vi "FPGA.vi"() -> ()   [LabVIEW 2013]
uses:
  <vilib>/rvi/FXPMathLib/FxpSinAndCos/XNode/nifxpmath_SinAndCos.xnode
  <vilib>/eio/EIONode/EIONode.xnode
  <vilib>/rvi/eio/common/nirviEmuTemplateMethod_errors.vi
  ToFPGA.ctl
  <vilib>/rvi/FXPMathLib/FxpSinAndCos/simVIs/DllFxpSinAndCosTemp_sub.vi
  <vilib>/rvi/FXPMathLib/FxpSinAndCos/subVIs/nifxpmath_SinAndCos_SimConfig.ctl
  FreqEstimator.ctl
  PMUmeasurements.ctl
panel:
  in  "Hold Time":sgl
  out "Loop period monitoring":u8
  out "output cluster":T1
  out "FPGA Error Out":errorcluster
  in  "alpha_Load":sgl
  in  "Scaling":sgl=80.0
  in  "Frequency Estimator Settings":T2={"Parameters"={"Ts"=5e-05, "kappaav"=0.625, "kappaph"=0.5762, "mu"=0.7086}}
  in  "Freq of Osc Load":sgl=0.64
  in  "PMU measurments":T3
  in  "stop":bool
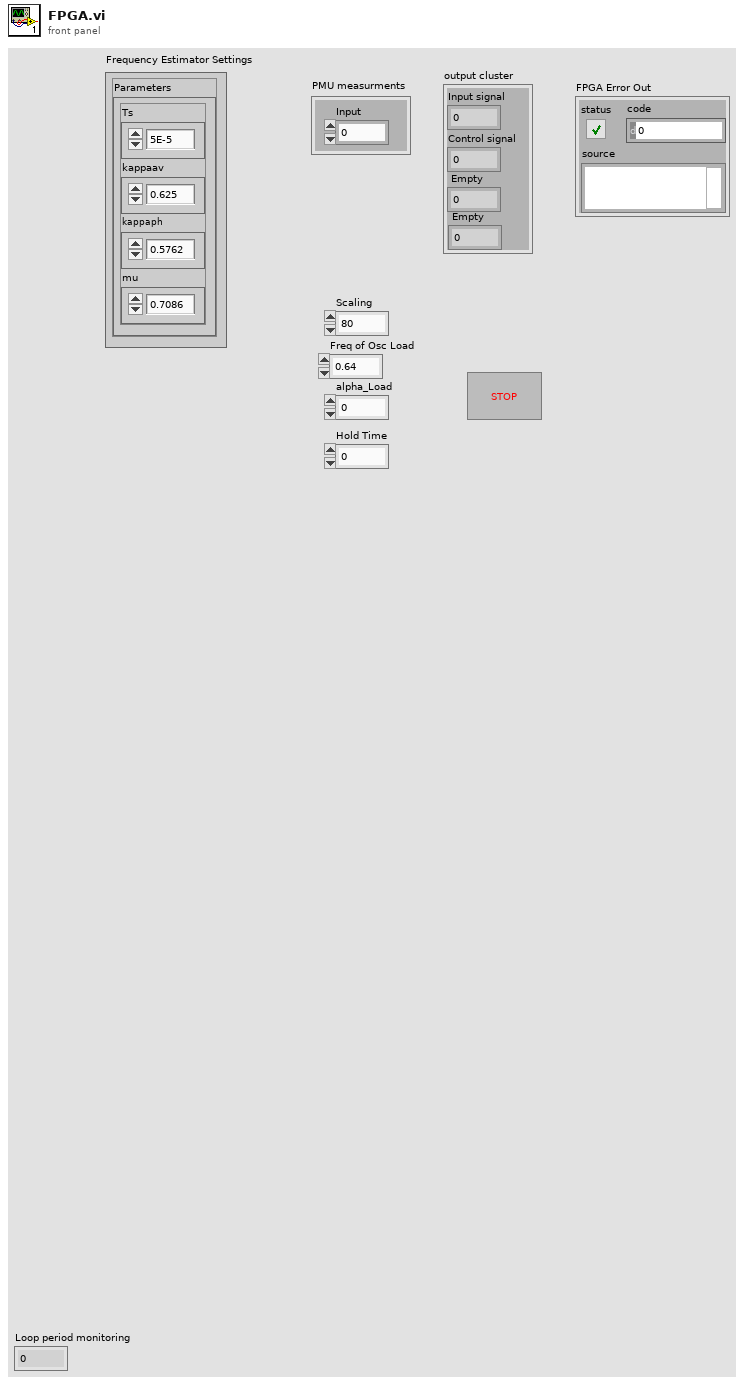
[diagram p1: front panel]
types:
  T1 = typedef "ToFPGA.ctl" = cluster{"Input signal":sgl, "Control signal":sgl, " Empty":sgl, " Empty":sgl}
  T2 = typedef "FreqEstimator.ctl" = cluster{"Parameters":cluster{"Ts":sgl, "kappaav":sgl, "kappaph":sgl, "mu":sgl}}
  T3 = typedef "PMUmeasurements.ctl" = cluster{"Input":sgl}
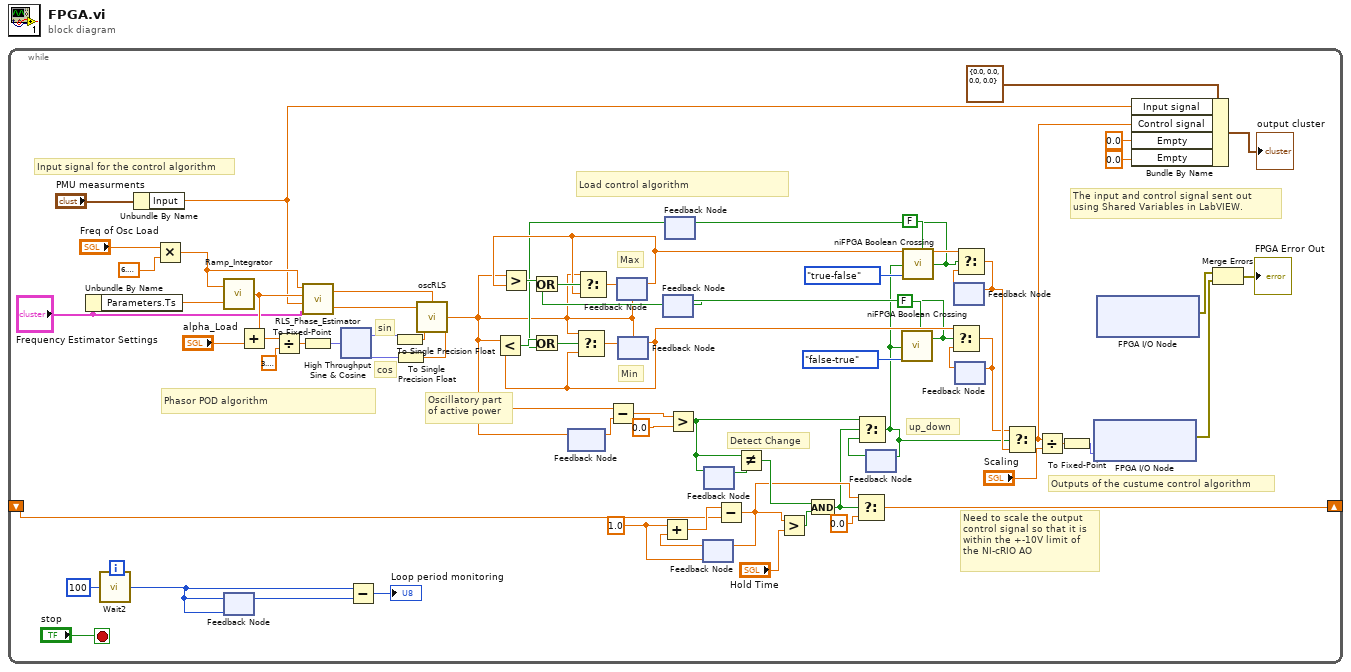
[diagram p0: block diagram]
diagram:
  n1 = while {
    shift-right: [w31] -> _
    shift-left: _ -> [w30]
    stop <- "stop" stop-if-true
    w37 = sgl 1.0 ("y")
    # "Need to scale the output \ncontrol signal so that it is \nwithin the +-10V limit of \nthe NI-cRIO AO"
    # "Load control algorithm"
    # "Phasor POD algorithm"
    # "Input signal for the control algorithm"
    # "The input and control signal sent out using Shared Variables in LabVIEW."
    # "Outputs of the custume control algorithm"
    # "up_down"
    # "Detect Change"
    # "Min"
    # "Max"
    # "Oscillatory part \nof active power"
    # "cos"
    # "sin"
    n2 = Unbundle By Name("Frequency Estimator Settings") -> ("Parameters.Ts"=w9:sgl)
    n3 = call "Wait2"("Count(uSec)"=u8 100) -> ("Tick Count(uSec)"=w41:u8)
    n4 = Unbundle By Name("PMU measurments") -> ("Input"=w7:sgl)
    n5 = Multiply(x="Freq of Osc Load", y=sgl 6.2831855) -> (x*y=w69:sgl)
    n6 = call "Ramp_Integrator.vi"("tsample"=w9, "w"=w69) -> ("theta"=w49:sgl)
    n7 = feedback #1(w41) -> (w42:u8)
    n8 = feedback-in #1(w41) -> ()
    n9 = Add(x=w49, y="alpha_Load") -> (x+y=w48:sgl)
    n10 = Divide(x=w48, y=sgl 3.1415927) -> (x/y=w67:sgl)
    n11 = call "RLS_Phase_Estimator.vi"("Frequency Estimator Settings"="Frequency Estimator Settings", "u"=w7, "theta"=w49, "wcs"=w69) -> ("uphq"=w60:sgl, "uphd"=w61:sgl)
    n12 = To Fixed-Point(number=w67) -> (fixed-point=w66:fxp<+/-,20,5>)  [unwired: 1 in]
    n13 = xnode "High Throughput Sine & Cosine"("x (pi)"=w66) -> ("sin(x)"=w65:fxp<+/-,16,2>, "cos(x)"=w64:fxp<+/-,16,2>)
    n14 = Subtract(x=w41, y=w42) -> (x-y=→"Loop period monitoring":u8)
    n15 = To Single Precision Float(number=w65) -> (single precision float=w63:sgl)
    n16 = To Single Precision Float(number=w64) -> (single precision float=w62:sgl)
    n17 = call "oscRLS.vi"("u4"=w63, "u3"=w62, "u2"=w60, "u1"=w61) -> ("f(u)"=w6:sgl)
    n18 = feedback #2() -> (w55:sgl)  [unwired: 1 in]
    n19 = feedback-in #2(w6) -> ()
    n20 = Subtract(x=w6, y=w55) -> (x-y=w53:sgl)
    n21 = feedback #3(w6) -> (w25:sgl)
    n22 = Greater?(x=w6, y=w25) -> (0:w59:bool)
    n23 = feedback #4(w6) -> (w24:sgl)
    n24 = Less?(x=w6, y=w24) -> (x < y?=w57:bool)
    n25 = feedback #5() -> (w16:bool)  [unwired: 1 in]
    n26 = Or(x=w59, y=w16) -> (x .or. y?=w58:bool)
    n27 = Select(t=w6, s=w58, f=w25) -> (s? t:f=w39:sgl)
    n28 = feedback-in #3(w39) -> ()
    n29 = feedback #6() -> (w18:bool)  [unwired: 1 in]
    n30 = Or(x=w57, y=w18) -> (x .or. y?=w56:bool)
    n31 = Select(t=w6, s=w56, f=w24) -> (s? t:f=w40:sgl)
    n32 = feedback-in #4(w40) -> ()
    n33 = Greater?(x=w53, y=sgl 0.0) -> (0:w29:bool)
    n34 = feedback #7(w37) -> (w38:sgl)
    n35 = Add(x=w37, y=w38) -> (x+y=w32:sgl)
    n36 = feedback #8(w29) -> (w34:bool)
    n37 = feedback-in #8(w29) -> ()
    n38 = Subtract(x=w32, y=w30) -> (x-y=w13:sgl)
    n39 = feedback-in #7(w13) -> ()
    n40 = Not Equal?(x=w29, y=w34) -> (x != y?=w14:bool)
    n41 = Greater?(x=w13, y="Hold Time") -> (0:w36:bool)
    n42 = And(x=w14, y=w36) -> (x .and. y?=w11:bool)
    n43 = Select(t=w13, s=w11, f=sgl 0.0) -> (s? t:f=w31:sgl)
    n44 = feedback #9() -> (w28:bool)  [unwired: 1 in]
    n45 = Select(t=w29, s=w11, f=w28) -> (s? t:f=w12:bool)
    n46 = feedback-in #9(w12) -> ()
    n47 = call <vilib>:"niFPGA Boolean Crossing.vi"("input"=w12, "direction"=enum8{"either", "false-true", "true-false"}."false-true", "initialize"=FALSE) -> ("crossing"=w17:bool)  [unwired: 6 in]
    n48 = feedback-in #5(w17) -> ()
    n49 = call <vilib>:"niFPGA Boolean Crossing.vi"("input"=w12, "direction"=enum8{"either", "false-true", "true-false"}."true-false", "initialize"=FALSE) -> ("crossing"=w19:bool)  [unwired: 6 in]
    n50 = feedback-in #6(w19) -> ()
    n51 = feedback #10() -> (w27:sgl)  [unwired: 1 in]
    n52 = feedback #11() -> (w26:sgl)  [unwired: 1 in]
    n53 = Select(t=w24, s=w17, f=w26) -> (s? t:f=w10:sgl)
    n54 = feedback-in #11(w10) -> ()
    n55 = Select(t=w25, s=w19, f=w27) -> (s? t:f=w15:sgl)
    n56 = feedback-in #10(w15) -> ()
    n57 = Select(t=w10, s=w12, f=w15) -> (s? t:f=w2:sgl)
    n58 = Divide(x=w2, y="Scaling") -> (x/y=w5:sgl)
    n59 = To Fixed-Point(number=w5) -> (fixed-point=w52:fxp<+/-,20,5>)  [unwired: 1 in]
    n60 = xnode "FPGA I/O Node"("Mod1/AO0"=w52) -> ("error out"=w46:errorcluster)  [unwired: 2 in, 1 out]
    n61 = xnode "FPGA I/O Node"() -> ("error out"=w47:errorcluster)  [unwired: 3 in, 1 out]
    n62 = Bundle By Name(cluster=T1 {"Input signal"=0.0, "Control signal"=0.0, " Empty"=0.0, " Empty"=0.0}, "Input signal"=w7, "Control signal"=w2, "Empty"=sgl 0.0, "Empty"=sgl 0.0) -> (→"output cluster":T1)
    n63 = Merge Errors(w47, w46) -> (→"FPGA Error Out":errorcluster)
  }
